vi "GetSensorValues.vi"(1 "Ref_LeftDriveEncoder":T3={"DeviceStatus"={"status"=FALSE, "code"=0, "source"=""}, "Type"=enum."PWM", "PWM"={"PWM Channel"=enum."Invalid", "DeadBand"={"Name"="", "maxPositivePwm"=0, "minPositivePwm"=0, "centerPwm"=0, "maxNegativePwm"=0, "minNegativePwm"=0, "angularRange"=0}}, "CAN"={"Device Number"=0, "SetOutput VI Ref"=variant, "GetOutput VI Ref"=variant, "Enable VI Ref"=variant, "Disable VI Ref"=variant, "Data"=variant}, "Invert"=FALSE, "DIO PWM"={"PWM \"Enable\" Channel"=enum."Invalid", "DIOChannel"=enum."Invalid", "PWM Rate"=0.0}}, 2 "Ref_RightDriveEncoder":T3={"DeviceStatus"={"status"=FALSE, "code"=0, "source"=""}, "Type"=enum."PWM", "PWM"={"PWM Channel"=enum."Invalid", "DeadBand"={"Name"="", "maxPositivePwm"=0, "minPositivePwm"=0, "centerPwm"=0, "maxNegativePwm"=0, "minNegativePwm"=0, "angularRange"=0}}, "CAN"={"Device Number"=0, "SetOutput VI Ref"=variant, "GetOutput VI Ref"=variant, "Enable VI Ref"=variant, "Disable VI Ref"=variant, "Data"=variant}, "Invert"=FALSE, "DIO PWM"={"PWM \"Enable\" Channel"=enum."Invalid", "DIOChannel"=enum."Invalid", "PWM Rate"=0.0}}, 3 "Rear Prox Sensor":T1, 4 "Right Prox Sensor":T1, 5 "Left Prox Sensor":T1, 6 "Upper Pressure Transducer":T1, 8 "Ref_Compressor":T8, 9 "Front-Right Prox Sensor":T1, 10 "Ref_ElevatorEncoder":T3={"DeviceStatus"={"status"=FALSE, "code"=0, "source"=""}, "Type"=enum."PWM", "PWM"={"PWM Channel"=enum."Invalid", "DeadBand"={"Name"="", "maxPositivePwm"=0, "minPositivePwm"=0, "centerPwm"=0, "maxNegativePwm"=0, "minNegativePwm"=0, "angularRange"=0}}, "CAN"={"Device Number"=0, "SetOutput VI Ref"=variant, "GetOutput VI Ref"=variant, "Enable VI Ref"=variant, "Disable VI Ref"=variant, "Data"=variant}, "Invert"=FALSE, "DIO PWM"={"PWM \"Enable\" Channel"=enum."Invalid", "DIOChannel"=enum."Invalid", "PWM Rate"=0.0}}, 11 "Front-Left Prox Sensor":T1, 13 "Lower Pressure Transducer":T1, 15 "Tank Pressure Transducer":T1) -> ()   [LabVIEW 2018]
uses:
  <vilib>/Rock Robotics/WPI/MotorControl/WPI_MotorControlDeviceRef.ctl
  <vilib>/Rock Robotics/WPI/MotorControl/WPI_MotorControlType.ctl
  <vilib>/Rock Robotics/SystemInterfaces/DIO/FPGA_DIOPWMChannel.ctl
  <vilib>/Rock Robotics/WPI/PWM/WPI_PWMDeadband.ctl
  <vilib>/Rock Robotics/SystemInterfaces/DIO/FPGA_DIOChannel.ctl
  <vilib>/Rock Robotics/WPI/AnalogChannel/WPI_AnalogChannelDevRef.ctl
  <vilib>/Rock Robotics/SystemInterfaces/AI/FPGA_AIChannel.ctl
  <vilib>/Rock Robotics/WPI/Compressor/WPI_CompressorDevRef.ctl
  SensorReadings.vi
  RobotStates.vi
  <vilib>/Rock Robotics/WPI/ThirdParty/Phoenix-LabVIEW/Motor Controller/Get/CTRE_Phoenix_MotorController_GetLimitSwitchStates.vi
  Inputs_DriverStation.vi
  RefNums_Actuators.vi
  <vilib>/Rock Robotics/WPI/ThirdParty/Phoenix-LabVIEW/Motor Controller/Get/CTRE_Phoenix_MotorController_GetSelectedSensorData.vi
  <vilib>/gmath/NI_Gmath.lvlib
panel:
  in  "Plot Drive Encoder Data":bool
  in  "Tank Pressure Voltage Table":dbl[](array[numeric])=[0.4, 0.7, 0.9, 1.2, 1.4, 1.7, 1.9, 2.3, 2.5, 2.8, 3.0, 3.3] format="%_6g"
  in  "Tank Pressure PSI Table":dbl[](array[numeric])=[0.0, 10.0, 20.0, 30.0, 40.0, 50.0, 60.0, 70.0, 80.0, 90.0, 100.0, 115.0] format="%_6g"
  in  "LR Voltage Table":dbl[](array[numeric])=[0.43, 0.45, 0.47, 0.55, 0.6, 0.68, 0.72, 0.81, 0.86, 0.98, 1.13, 1.36, 1.53, 1.77, 1.99, 2.26, 2.52, 2.76] format="%_6g"
  in  "LR Distance Table":dbl[](array[numeric])=[150.661, 140.6, 133.7, 120.9, 110.1, 95.3, 90.1, 80.0, 73.7, 64.6, 55.9, 45.6, 40.2, 35.0, 29.6, 24.3, 19.6, 14.8] format="%_6g"
  in  "Suction Threshold (V)":dbl=0.2
  in  "SR Voltage Table":dbl[](array[numeric])=[3.15, 2.82, 2.51, 2.16, 1.92, 1.7, 1.49, 1.3, 1.12, 0.97, 0.87, 0.79, 0.72, 0.64, 0.61, 0.58, 0.52, 0.47, 0.46, 0.45, 0.43, 0.41] format="%_6g"
  in  "SR Distance Table":dbl[](array[numeric])=[4.6, 6.6, 8.3, 10.4, 12.2, 14.1, 16.5, 19.9, 23.6, 28.2, 32.6, 36.8, 40.9, 46.3, 49.9, 53.7, 58.3, 63.5, 67.5, 71.5, 75.1, 78.9] format="%_6g"
  out "Drive Encoder Positions":cluster{dbl, dbl}(graph)
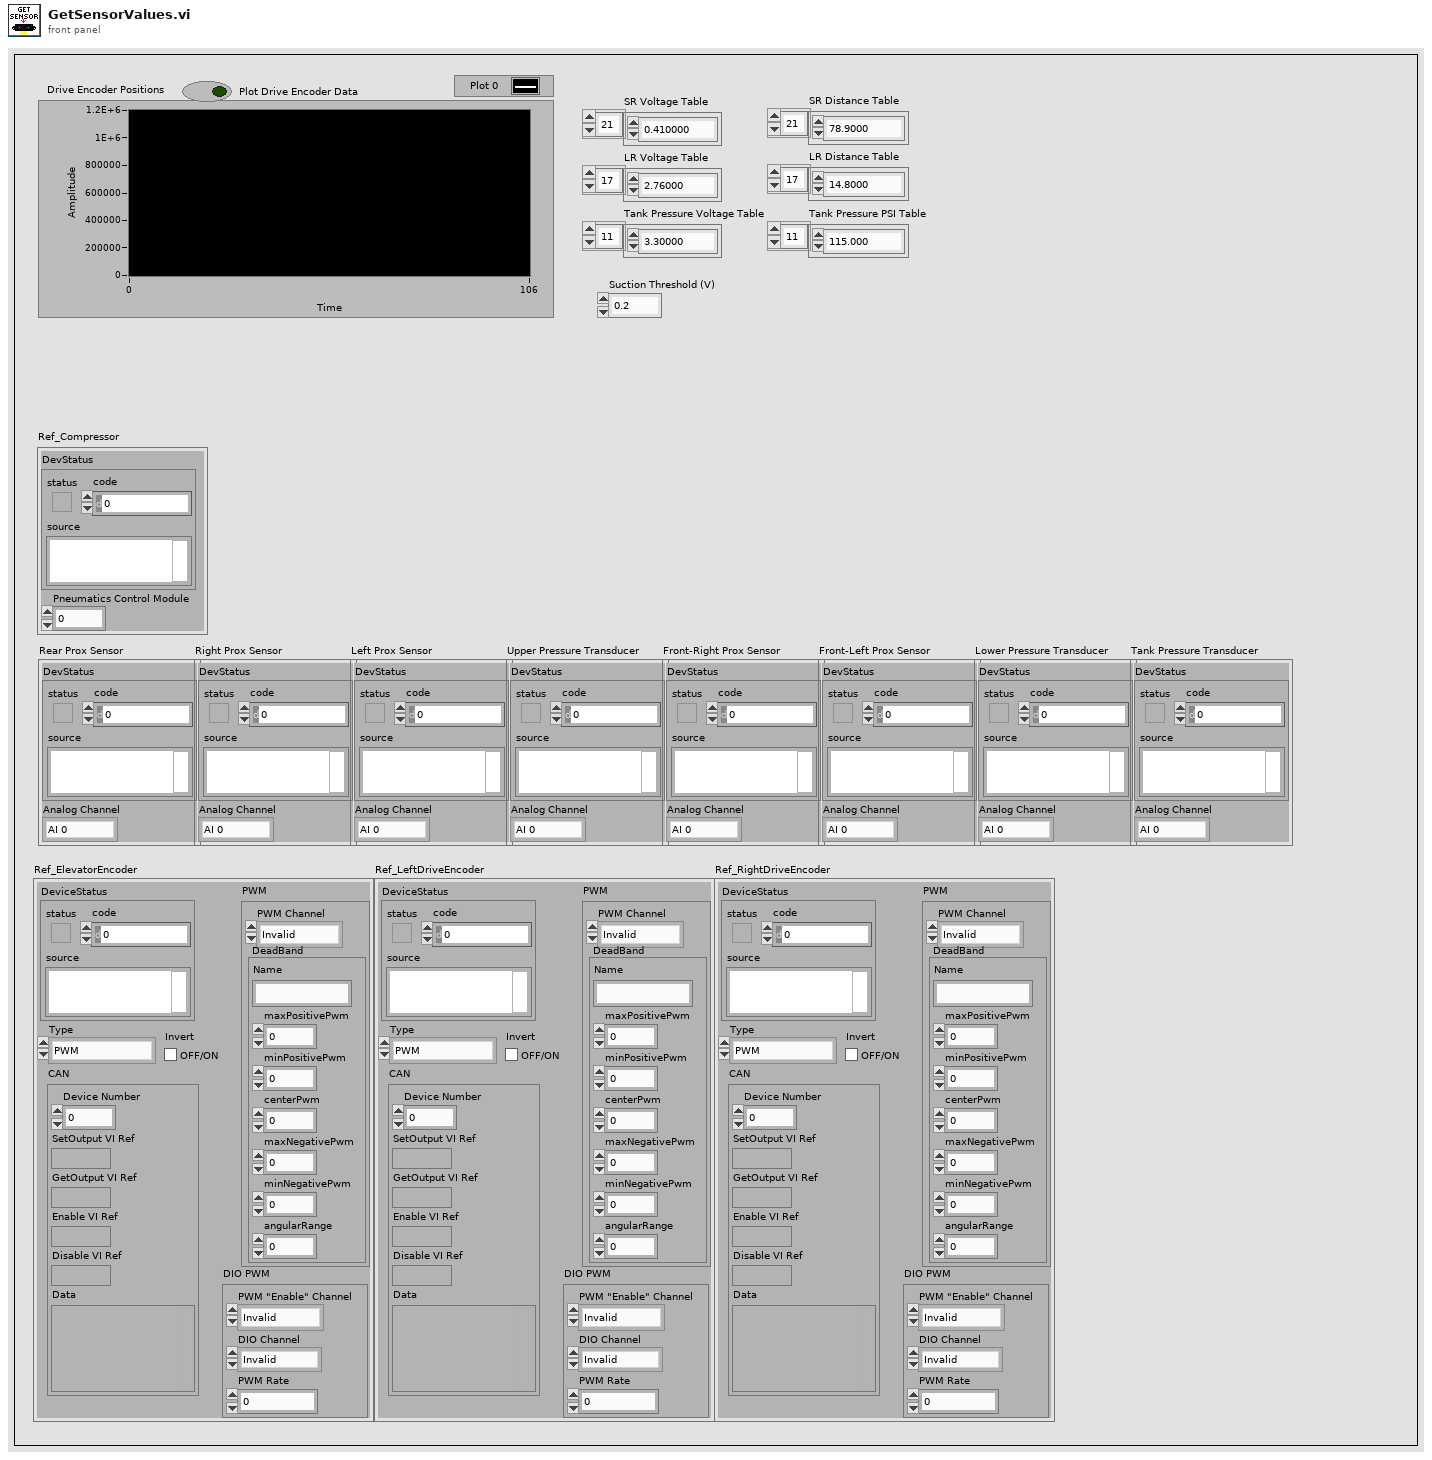
[diagram p1: front panel]
types:
  T1 = typedef "WPI_AnalogChannelDevRef.ctl" = cluster{"DevStatus":errorcluster, "Analog Channel":T2}
  T2 = typedef "FPGA_AIChannel.ctl" = enum8{"AI 0", "AI 1", "AI 2", "AI 3", "AI MXP 0", "AI MXP 1", "AI MXP 2", "AI MXP 3", "Invalid"}
  T3 = typedef "WPI_MotorControlDeviceRef.ctl" = cluster{"DeviceStatus":errorcluster, "Type":T4, "PWM":cluster{"PWM Channel":T5, "DeadBand":T6}, "CAN":cluster{"Device Number":u8, "SetOutput VI Ref":variant, "GetOutput VI Ref":variant, "Enable VI Ref":variant, "Disable VI Ref":variant, "Data":variant}, "Invert":bool, "DIO PWM":cluster{"PWM \"Enable\" Channel":T5, "DIOChannel":T7, "PWM Rate":dbl}}
  T4 = typedef "WPI_MotorControlType.ctl" = enum16{"PWM", "CAN", "DIO PWM"}
  T5 = typedef "FPGA_DIOPWMChannel.ctl" = enum8{"PWM 0", "PWM 1", "PWM 2", "PWM 3", "PWM 4", "PWM 5", "PWM 6", "PWM 7", "PWM 8", "PWM 9", "PWM MXP 0", "PWM MXP 1", "PWM MXP 2", "PWM MXP 3", "PWM MXP 4", "PWM MXP 5", "PWM MXP 6", "PWM MXP 7", "PWM MXP 8", "PWM MXP 9", "Invalid"}
  T6 = typedef "WPI_PWMDeadband.ctl" = cluster{"Name":string, "maxPositivePwm":i32, "minPositivePwm":i32, "centerPwm":i32, "maxNegativePwm":i32, "minNegativePwm":i32, "angularRange":u16}
  T7 = typedef "FPGA_DIOChannel.ctl" = enum8{"DIO 0", "DIO 1", "DIO 2", "DIO 3", "DIO 4", "DIO 5", "DIO 6", "DIO 7", "DIO 8", "DIO 9", "DIO MXP 0", "DIO MXP 1", "DIO MXP 2", "DIO MXP 3", "DIO MXP 4", "DIO MXP 5", "DIO MXP 6", "DIO MXP 7", "DIO MXP 8", "DIO MXP 9", "DIO MXP 10", "DIO MXP 11", "DIO MXP 12", "DIO MXP 13", "DIO MXP 14", "DIO MXP 15", "SPI Port CS1", "SPI Port CS2", "SPI Port CS3", "SPI Port MISO", "SPI Port MOSI", "Invalid"}
  T8 = typedef "WPI_CompressorDevRef.ctl" = cluster{"DevStatus":errorcluster, "Pneumatics Control Module":u8}
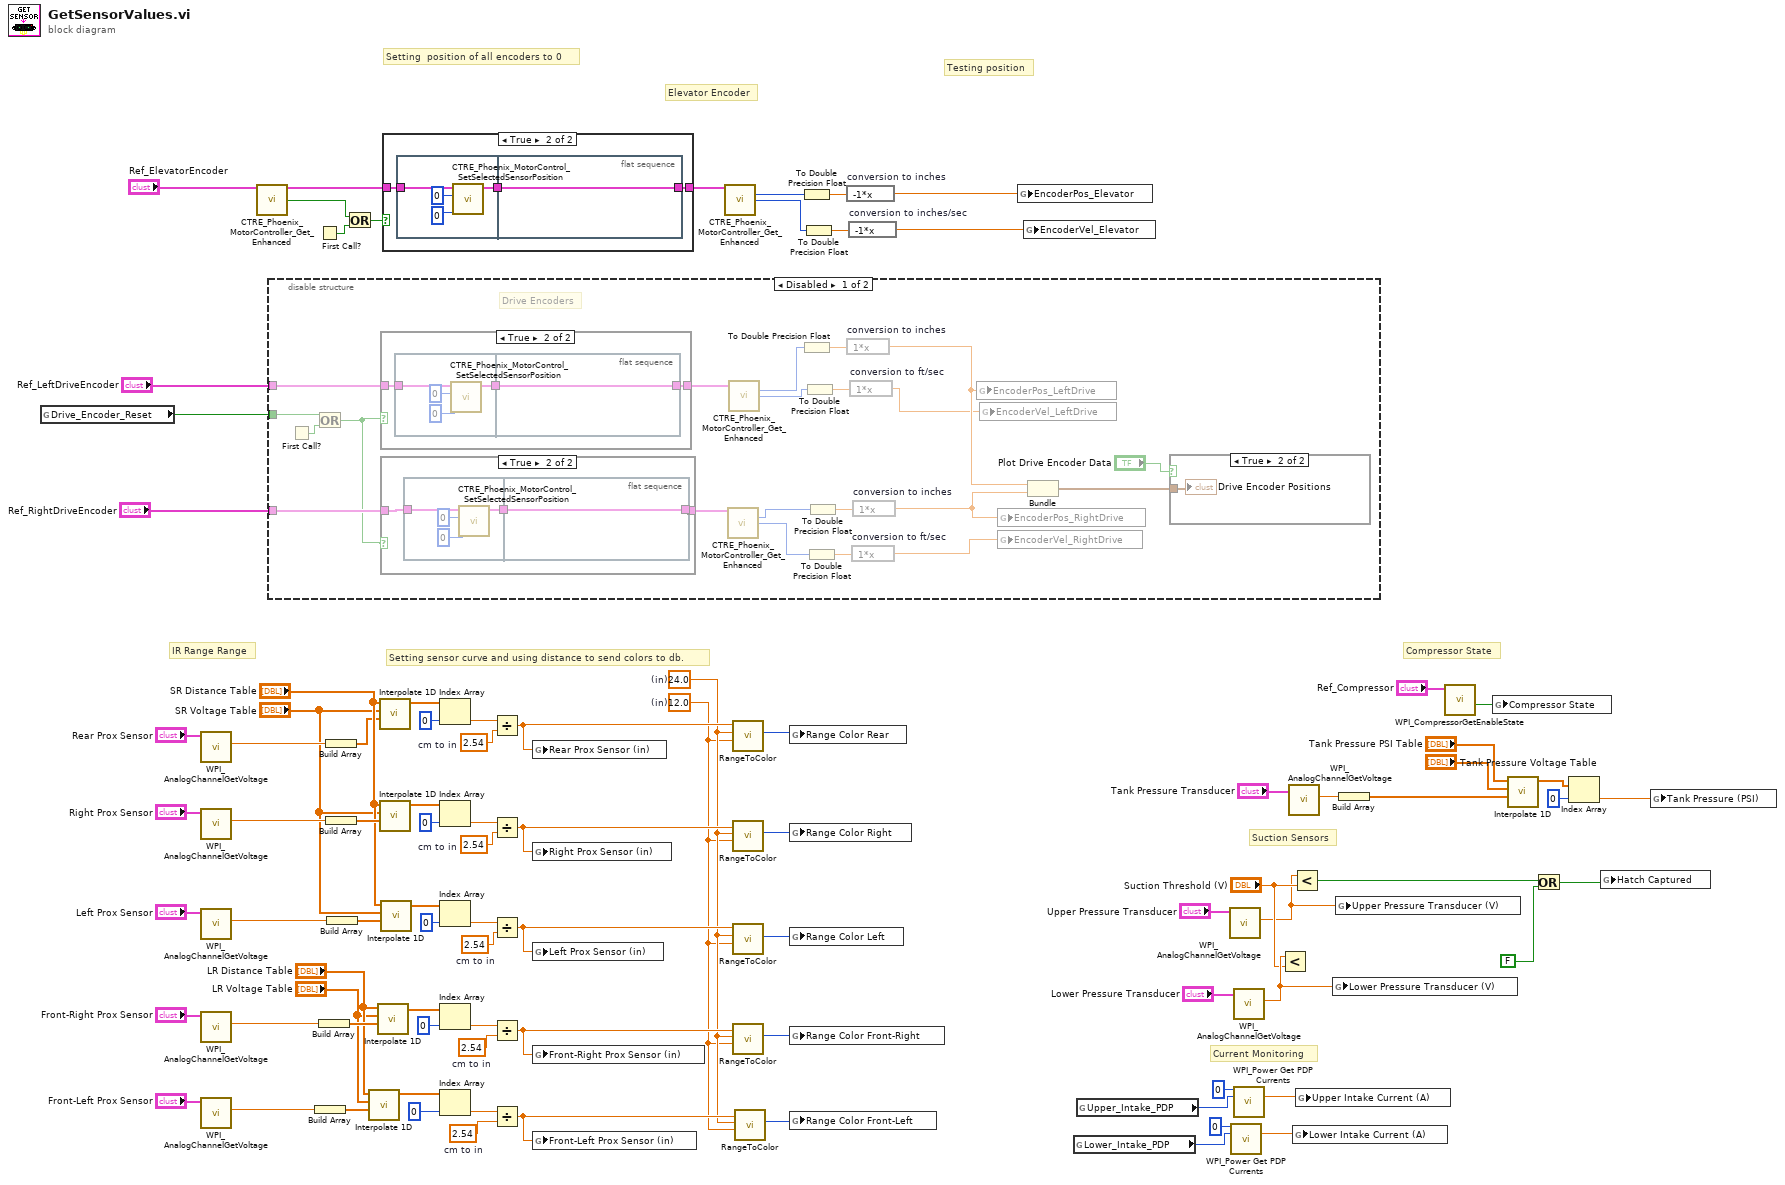
[diagram p0: block diagram]
diagram:
  w40 = 2.54  # cm to in
  w30 = 12.0  # (in)
  w31 = 24.0  # (in)
  w64 = 2.54  # cm to in
  w70 = 2.54  # cm to in
  w77 = 2.54  # cm to in
  w84 = 2.54  # cm to in
  # "Testing position"
  # "Setting  position of all encoders to 0"
  # "Setting sensor curve and using distance to send colors to db."
  # "Current Monitoring"
  # "Suction Sensors"
  # "Elevator Encoder"
  # "Compressor State"
  # "IR Range Range"
  n1 = global read "Inputs_DriverStation.vi" "Drive_Encoder_Reset"() -> (w21:bool)
  n2 = call <vilib>:"WPI_AnalogChannelGetVoltage.vi"("AIDeviceRef"="Rear Prox Sensor") -> ("Voltage"=w88:dbl)  [unwired: 8 in, 2 out]
  n3 = call <vilib>:"WPI_AnalogChannelGetVoltage.vi"("AIDeviceRef"="Right Prox Sensor") -> ("Voltage"=w82:dbl)  [unwired: 8 in, 2 out]
  n4 = call <vilib>:"WPI_AnalogChannelGetVoltage.vi"("AIDeviceRef"="Left Prox Sensor") -> ("Voltage"=w75:dbl)  [unwired: 8 in, 2 out]
  n5 = call <vilib>:"WPI_AnalogChannelGetVoltage.vi"("AIDeviceRef"="Front-Right Prox Sensor") -> ("Voltage"=w45:dbl)  [unwired: 8 in, 2 out]
  n6 = call <vilib>:"WPI_AnalogChannelGetVoltage.vi"("AIDeviceRef"="Front-Left Prox Sensor") -> ("Voltage"=w38:dbl)  [unwired: 8 in, 2 out]
  n7 = call-poly <vilib>:"CTRE_Phoenix_MotorController_Get_Enhanced.vi"("PhoenixMotorControlDevRef"="Ref_ElevatorEncoder") -> ("PhoenixMotorControlDevRef"=w13:T3, "Reverse Limit Closed?"=w11:bool)  [unwired: 11 in, 2 out]
  n8 = disable-structure shown="Disabled" {
    disable-tunnel: "Ref_LeftDriveEncoder" -> [w111 _]
    disable-tunnel: "Ref_RightDriveEncoder" -> [w110 _]
    disable-tunnel: w21 -> [w109 _]
    frame Disabled {
      # "Drive Encoders"
      n9 = First Call?() -> (First Call?: T/F=w93:bool)
      n10 = Or(x=w109, y=w93) -> (x .or. y?=w92:bool)
      n11 = case shown="True" w92 {
        tunnel: w111 -> [w122 w125]
        tunnel: [w122 w123] -> w108
        frame False {
        }
        frame True {
          n12 = flat-sequence {
            tunnel: w125 -> [w129]
            tunnel: [w128] -> w124
            tunnel: [w130] -> w123
            tunnel: w124 -> [w130]
            frame #0 {
              n13 = call <vilib>:"CTRE_Phoenix_MotorControl_SetSelectedSensorPosition.vi"("pidLoopIdx"=u32 0, "New Sensor Position"=0, "PhoenixMotorControlDevRef"=w129) -> ("PhoenixMotorControlDevRef"=w128:T3)  [unwired: 7 in, 1 out]
            }
            frame #1 {
            }
          }
        }
      }
      n14 = case shown="True" w92 {
        tunnel: w110 -> [w113 w116]
        tunnel: [w113 w114] -> w107
        frame False {
        }
        frame True {
          n15 = flat-sequence {
            tunnel: w116 -> [w120]
            tunnel: [w119] -> w115
            tunnel: [w121] -> w114
            tunnel: w115 -> [w121]
            frame #0 {
              n16 = call <vilib>:"CTRE_Phoenix_MotorControl_SetSelectedSensorPosition.vi"("pidLoopIdx"=u32 0, "New Sensor Position"=0, "PhoenixMotorControlDevRef"=w120) -> ("PhoenixMotorControlDevRef"=w119:T3)  [unwired: 7 in, 1 out]
            }
            frame #1 {
            }
          }
        }
      }
      n17 = call-poly <vilib>:"CTRE_Phoenix_MotorController_Get_Enhanced.vi"("PhoenixMotorControlDevRef"=w107) -> ("Position (Raw Sensor Units)"=w98:i32, "Velocity (Raw Sensor Units per 100 ms)"=w95:i32)  [unwired: 11 in, 2 out]
      n18 = call-poly <vilib>:"CTRE_Phoenix_MotorController_Get_Enhanced.vi"("PhoenixMotorControlDevRef"=w108) -> ("Position (Raw Sensor Units)"=w105:i32, "Velocity (Raw Sensor Units per 100 ms)"=w101:i32)  [unwired: 11 in, 2 out]
      n19 = To Double Precision Float(number=w105) -> (double precision float=w104:dbl)
      n20 = To Double Precision Float(number=w101) -> (double precision float=w102:dbl)
      n21 = To Double Precision Float(number=w95) -> (double precision float=w96:dbl)
      n22 = To Double Precision Float(number=w98) -> (double precision float=w99:dbl)
      n23 = expression code="1*x" "conversion to inches"(w104) -> (w103:dbl)
      n24 = expression code="1*x" "conversion to ft/sec"(w102) -> (w100:dbl)
      n25 = expression code="1*x" "conversion to ft/sec"(w96) -> (w94:dbl)
      n26 = expression code="1*x" "conversion to inches"(w99) -> (w97:dbl)
      n27 = global write "SensorReadings.vi" "EncoderPos_LeftDrive"(w103) -> ()
      n28 = global write "SensorReadings.vi" "EncoderVel_LeftDrive"(w100) -> ()
      n29 = global write "SensorReadings.vi" "EncoderPos_RightDrive"(w97) -> ()
      n30 = global write "SensorReadings.vi" "EncoderVel_RightDrive"(w94) -> ()
      n31 = Bundle(w103, w97) -> (w106:cluster{dbl, dbl})  [unwired: 1 in]
      n32 = case shown="True" "Plot Drive Encoder Data" {
        tunnel: w106 -> [_ w112]
        frame False {
        }
        frame True {
          "Drive Encoder Positions" <- w112
        }
      }
    }
    frame Enabled {
    }
  }
  n33 = First Call?() -> (First Call?: T/F=w10:bool)
  n34 = Build Array(w38) -> (w43:dbl[])
  n35 = Build Array(w45) -> (w68:dbl[])
  n36 = Build Array(w88) -> (w61:dbl[])
  n37 = Build Array(w82) -> (w81:dbl[])
  n38 = Build Array(w75) -> (w74:dbl[])
  n39 = Or(x=w11, y=w10) -> (x .or. y?=w12:bool)
  n40 = call <vilib>:"Interpolate 1D.vi"("xi"=w43, "X"="LR Voltage Table", "Y"="LR Distance Table") -> ("yi"=w37:dbl[])  [unwired: 6 in, 2 out]
  n41 = call <vilib>:"Interpolate 1D.vi"("xi"=w68, "X"="LR Voltage Table", "Y"="LR Distance Table") -> ("yi"=w65:dbl[])  [unwired: 6 in, 2 out]
  n42 = call <vilib>:"Interpolate 1D.vi"("xi"=w61, "X"="SR Voltage Table", "Y"="SR Distance Table") -> ("yi"=w85:dbl[])  [unwired: 6 in, 2 out]
  n43 = call <vilib>:"Interpolate 1D.vi"("xi"=w81, "X"="SR Voltage Table", "Y"="SR Distance Table") -> ("yi"=w78:dbl[])  [unwired: 6 in, 2 out]
  n44 = call <vilib>:"Interpolate 1D.vi"("xi"=w74, "X"="SR Voltage Table", "Y"="SR Distance Table") -> ("yi"=w71:dbl[])  [unwired: 6 in, 2 out]
  n45 = case shown="True" w12 {
    tunnel: w13 -> [w131 w134]
    tunnel: [w131 w132] -> w19
    frame False {
    }
    frame True {
      n46 = flat-sequence {
        tunnel: w134 -> [w138]
        tunnel: [w137] -> w133
        tunnel: [w139] -> w132
        tunnel: w133 -> [w139]
        frame #0 {
          n47 = call <vilib>:"CTRE_Phoenix_MotorControl_SetSelectedSensorPosition.vi"("pidLoopIdx"=u32 0, "New Sensor Position"=0, "PhoenixMotorControlDevRef"=w138) -> ("PhoenixMotorControlDevRef"=w137:T3)  [unwired: 7 in, 1 out]
        }
        frame #1 {
        }
      }
    }
  }
  n48 = Index Array(array=w85, index=0) -> (element=w86:dbl)
  n49 = Index Array(array=w78, index=0) -> (element=w79:dbl)
  n50 = Index Array(array=w71, index=0) -> (element=w72:dbl)
  n51 = Index Array(array=w65, index=0) -> (element=w66:dbl)
  n52 = Index Array(array=w37, index=0) -> (element=w41:dbl)
  n53 = Divide(x=w86, y=w84) -> (x/y=w60:dbl)
  n54 = Divide(x=w79, y=w77) -> (x/y=w59:dbl)
  n55 = Divide(x=w72, y=w70) -> (x/y=w58:dbl)
  n56 = Divide(x=w66, y=w64) -> (x/y=w57:dbl)
  n57 = Divide(x=w41, y=w40) -> (x/y=w39:dbl)
  n58 = global write "SensorReadings.vi" "Rear Prox Sensor (in)"(w60) -> ()
  n59 = global write "SensorReadings.vi" "Right Prox Sensor (in)"(w59) -> ()
  n60 = global write "SensorReadings.vi" "Left Prox Sensor (in)"(w58) -> ()
  n61 = global write "SensorReadings.vi" "Front-Right Prox Sensor (in)"(w57) -> ()
  n62 = global write "SensorReadings.vi" "Front-Left Prox Sensor (in)"(w39) -> ()
  n63 = call-poly <vilib>:"CTRE_Phoenix_MotorController_Get_Enhanced.vi"("PhoenixMotorControlDevRef"=w19) -> ("Position (Raw Sensor Units)"=w18:i32, "Velocity (Raw Sensor Units per 100 ms)"=w16:i32)  [unwired: 11 in, 2 out]
  n64 = call "RangeToColor.vi"("Really Close (in)"=w30, "Close (in)"=w31, "Range (in)"=w60) -> ("Range Color"=w56:u32)  [unwired: 8 in]
  n65 = call "RangeToColor.vi"("Really Close (in)"=w30, "Close (in)"=w31, "Range (in)"=w59) -> ("Range Color"=w55:u32)  [unwired: 8 in]
  n66 = call "RangeToColor.vi"("Really Close (in)"=w30, "Close (in)"=w31, "Range (in)"=w58) -> ("Range Color"=w54:u32)  [unwired: 8 in]
  n67 = call "RangeToColor.vi"("Really Close (in)"=w30, "Close (in)"=w31, "Range (in)"=w57) -> ("Range Color"=w53:u32)  [unwired: 8 in]
  n68 = call "RangeToColor.vi"("Really Close (in)"=w30, "Close (in)"=w31, "Range (in)"=w39) -> ("Range Color"=w32:u32)  [unwired: 8 in]
  n69 = global write "SensorReadings.vi" "Range Color Rear"(w56) -> ()
  n70 = global write "SensorReadings.vi" "Range Color Right"(w55) -> ()
  n71 = global write "SensorReadings.vi" "Range Color Left"(w54) -> ()
  n72 = global write "SensorReadings.vi" "Range Color Front-Right"(w53) -> ()
  n73 = global write "SensorReadings.vi" "Range Color Front-Left"(w32) -> ()
  n74 = To Double Precision Float(number=w18) -> (double precision float=w20:dbl)
  n75 = To Double Precision Float(number=w16) -> (double precision float=w17:dbl)
  n76 = expression code="-1*x" "conversion to inches"(w20) -> (w14:dbl)
  n77 = expression code="-1*x" "conversion to inches/sec"(w17) -> (w15:dbl)
  n78 = global write "SensorReadings.vi" "EncoderPos_Elevator"(w14) -> ()
  n79 = global write "SensorReadings.vi" "EncoderVel_Elevator"(w15) -> ()
  n80 = global read "RefNums_Actuators.vi" "Lower_Intake_PDP"() -> (w25:i32)
  n81 = global read "RefNums_Actuators.vi" "Upper_Intake_PDP"() -> (w28:i32)
  n82 = call <vilib>:"WPI_AnalogChannelGetVoltage.vi"("AIDeviceRef"="Upper Pressure Transducer") -> ("Voltage"=w3:dbl)  [unwired: 8 in, 2 out]
  n83 = call <vilib>:"WPI_Power Get PDP Currents.vi"("Power Distribution Panel (0)"=u8 0, "PDP Channel"=w25) -> ("current (A)"=w24:dbl)  [unwired: 11 in, 2 out]
  n84 = call <vilib>:"WPI_AnalogChannelGetVoltage.vi"("AIDeviceRef"="Lower Pressure Transducer") -> ("Voltage"=w49:dbl)  [unwired: 8 in, 2 out]
  n85 = call <vilib>:"WPI_Power Get PDP Currents.vi"("Power Distribution Panel (0)"=u8 0, "PDP Channel"=w28) -> ("current (A)"=w27:dbl)  [unwired: 11 in, 2 out]
  n86 = Less?(x=w49, y="Suction Threshold (V)") -> ()  [unwired: 1 out]
  n87 = call <vilib>:"WPI_AnalogChannelGetVoltage.vi"("AIDeviceRef"="Tank Pressure Transducer") -> ("Voltage"=w1:dbl)  [unwired: 8 in, 2 out]
  n88 = Less?(x=w3, y="Suction Threshold (V)") -> (x < y?=w47:bool)
  n89 = global write "SensorReadings.vi" "Lower Intake Current (A)"(w24) -> ()
  n90 = global write "SensorReadings.vi" "Upper Intake Current (A)"(w27) -> ()
  n91 = global write "SensorReadings.vi" "Lower Pressure Transducer (V)"(w49) -> ()
  n92 = global write "SensorReadings.vi" "Upper Pressure Transducer (V)"(w3) -> ()
  n93 = Build Array(w1) -> (w5:dbl[])
  n94 = call <vilib>:"WPI_CompressorGetEnableState.vi"("CompressorDevRef"="Ref_Compressor") -> ("Compressor Running"=w50:bool)  [unwired: 7 in, 3 out]
  n95 = global write "RobotStates.vi" "Compressor State"(w50) -> ()
  n96 = call <vilib>:"Interpolate 1D.vi"("xi"=w5, "X"="Tank Pressure Voltage Table", "Y"="Tank Pressure PSI Table") -> ("yi"=w8:dbl[])  [unwired: 6 in, 2 out]
  n97 = Or(x=w47, y=FALSE) -> (x .or. y?=w4:bool)
  n98 = Index Array(array=w8, index=0) -> (element=w2:dbl)
  n99 = global write "SensorReadings.vi" "Hatch Captured"(w4) -> ()
  n100 = global write "SensorReadings.vi" "Tank Pressure (PSI)"(w2) -> ()
